vi "Begin.vi"(8 "error in":errorcluster) -> (0 "error out":errorcluster)   [LabVIEW 2015]
doc: "Called before other user functions, this VI is expected to open initial I/O refnums, load in file data, and do all program initialization. Notice that the <B>error out</B> terminal is simply used for data flow. Wiring it to other structures or subVIs ensures that this VI runs first."
uses:
  <vilib>/Rock Robotics/WPI/DriverStation/WPI_DriverStationRobotMode2.ctl
  <vilib>/Rock Robotics/WPI/Joystick/WPI_JoystickDeviceEnum.ctl
  <vilib>/Rock Robotics/SystemInterfaces/DIO/FPGA_DIOChannel.ctl
  <vilib>/Rock Robotics/WPI/Solenoid/WPI_SolenoidChannel.ctl
  Robot Global Data.vi
  <vilib>/Rock Robotics/Network Tables/NT Write String Array.vi
  <vilib>/Rock Robotics/WPI/RobotDrive/WPI_RobotDriveOpen2MotorWithCANTalonSRX.vi
  <vilib>/Rock Robotics/WPI/Utilities/WPI_GetSetVariantRefNum.vi
  <vilib>/Rock Robotics/WPI/MotorControl/WPI_MotorControlOpenCANTalonSRX.vi
  <vilib>/Rock Robotics/WPI/Solenoid/WPI_SolenoidOpenSingle.vi
  <vilib>/Rock Robotics/WPI/Solenoid/WPI_SolenoidOpenDouble.vi
  <vilib>/Rock Robotics/WPI/RobotDrive/WPI_RobotDriveOpen4MotorWithCANTalonSRX.vi
  <vilib>/Rock Robotics/WPI/Accelerometer/InternalAccelerometer/WPI_AccelerometerInternalOpen.vi
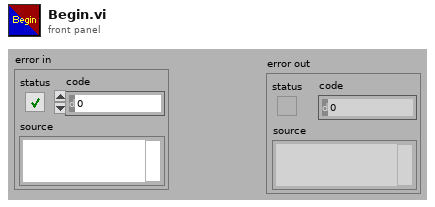
[diagram p1: front panel]
types:
  T1 = typedef "WPI_SolenoidChannel.ctl" = enum8{"Solenoid 0", "Solenoid 1", "Solenoid 2", "Solenoid 3", "Solenoid 4", "Solenoid 5", "Solenoid 6", "Solenoid 7", "Invalid"}
  T2 = typedef "FPGA_DIOChannel.ctl" = enum8{"DIO 0", "DIO 1", "DIO 2", "DIO 3", "DIO 4", "DIO 5", "DIO 6", "DIO 7", "DIO 8", "DIO 9", "DIO MXP 0", "DIO MXP 1", "DIO MXP 2", "DIO MXP 3", "DIO MXP 4", "DIO MXP 5", "DIO MXP 6", "DIO MXP 7", "DIO MXP 8", "DIO MXP 9", "DIO MXP 10", "DIO MXP 11", "DIO MXP 12", "DIO MXP 13", "DIO MXP 14", "DIO MXP 15", "Invalid"}
  T3 = typedef "WPI_JoystickDeviceEnum.ctl" = enum16{"USB 0", "USB 1", "USB 2", "USB 3", "USB 4", "USB 5"}
  T4 = typedef "WPI_DriverStationRobotMode2.ctl" = enum16{"Autonomous Disabled", "Autonomous Enabled", "Teleop Disabled", "Teleop Enabled", "Disconnected", "Finish", "Test Disabled", "Test Enabled", "Emergency Stopped"}
  T5 = typedef "WPI_AccelerometerDevRef.ctl" = cluster{"DevStatus":errorcluster, "Scaling":T6, "Analog Channels":T7, "I2C Bus":T9, "SPI Bus":T10, "Accel Range":T11, "ADXL Axes":T12, "Handle":i32, "Device Address":u8, "Accel Type":enum16{"Analog", "ADXL345 I2C", "ADXL345 SPI", "Internal", "ADXL362 SPI"}}
  T6 = typedef "WPI_AccelerometerScaling.ctl" = cluster{"Gain (VoltsPerG)":dbl, "Center Voltage":dbl}
  T7 = typedef "WPI_AccelerometerAnalogChannels.ctl" = cluster{"X-Axis":T8, "Y-Axis":T8, "Z-Axis":T8}
  T8 = typedef "FPGA_AIChannel.ctl" = enum8{"AI 0", "AI 1", "AI 2", "AI 3", "AI MXP 0", "AI MXP 1", "AI MXP 2", "AI MXP 3", "Invalid"}
  T9 = typedef "i2c_bus.ctl" = enum16{"I2C On-Board", "I2C MXP", "Invalid"}
  T10 = typedef "spi_bus.ctl" = enum16{"SPI On-Board, CS0", "SPI On-Board, CS1", "SPI On-Board, CS2", "SPI On-Board, CS3", "SPI MXP", "Invalid"}
  T11 = typedef "ADXL345 Range.ctl" = u8
  T12 = typedef "WPI_AccelerometerADXL345 Axes.ctl" = cluster{"X-Axis":bool, "Y-Axis":bool, "Z-Axis":bool}
  T13 = typedef "WPI_CompressorDevRef.ctl" = cluster{"DevStatus":errorcluster, "Pneumatics Control Module":u8}
  T14 = typedef "WPI_RobotDriveDevRef.ctl" = cluster{"DevStatus":errorcluster, "Motors[]":T15[], "Square Inputs":bool, "Max Output":dbl}
  T15 = typedef "WPI_MotorControlDeviceRef.ctl" = cluster{"DeviceStatus":errorcluster, "Type":T16, "PWM":cluster{"PWM Channel":T17, "DeadBand":T18}, "CAN":cluster{"Device Number":u8, "Control Mode":T19, "Semaphore":T20, "Max Vout":dbl, "TalonSRX Control Mode":T21}, "Invert":bool}
  T16 = typedef "WPI_MotorControlType.ctl" = enum16{"PWM", "CAN", "CANTalonSRX"}
  T17 = typedef "FPGA_DIOPWMChannel.ctl" = enum8{"PWM 0", "PWM 1", "PWM 2", "PWM 3", "PWM 4", "PWM 5", "PWM 6", "PWM 7", "PWM 8", "PWM 9", "PWM MXP 0", "PWM MXP 1", "PWM MXP 2", "PWM MXP 3", "PWM MXP 4", "PWM MXP 5", "PWM MXP 6", "PWM MXP 7", "PWM MXP 8", "PWM MXP 9", "Invalid"}
  T18 = typedef "WPI_PWMDeadband.ctl" = cluster{"Name":string, "maxPositivePwm":i32, "minPositivePwm":i32, "centerPwm":i32, "maxNegativePwm":i32, "minNegativePwm":i32, "angularRange":u16}
  T19 = typedef "WPI_CANJaguar_ControlMode.ctl" = enum8{"Percent VBus", "Current", "Speed", "Position", "Voltage"}
  T20 = typedef "Semaphore RefNum" = refnum<k1>
  T21 = typedef "WPI_CANTalonSRX_APIControlMode.ctl" = enum8{"Percent VBus", "Speed", "Position", "Slave", "Unchanged / Invalid", "Voltage Compensation", "Current", "Motion Profile"}
  T22 = typedef "WPI_JoystickDevRef.ctl" = cluster{"Device":T3}
  T23 = typedef "WPI_DigitalInputDevRef.ctl" = cluster{"DevStatus":errorcluster, "DIO Channel":T2}
  T24 = typedef "WPI_SolenoidDevRef.ctl" = cluster{"DevStatus":errorcluster, "Pneumatics Control Module":u8, "Forward Solenoid Channel":T1, "Reverse Solenoid Channel":T1}
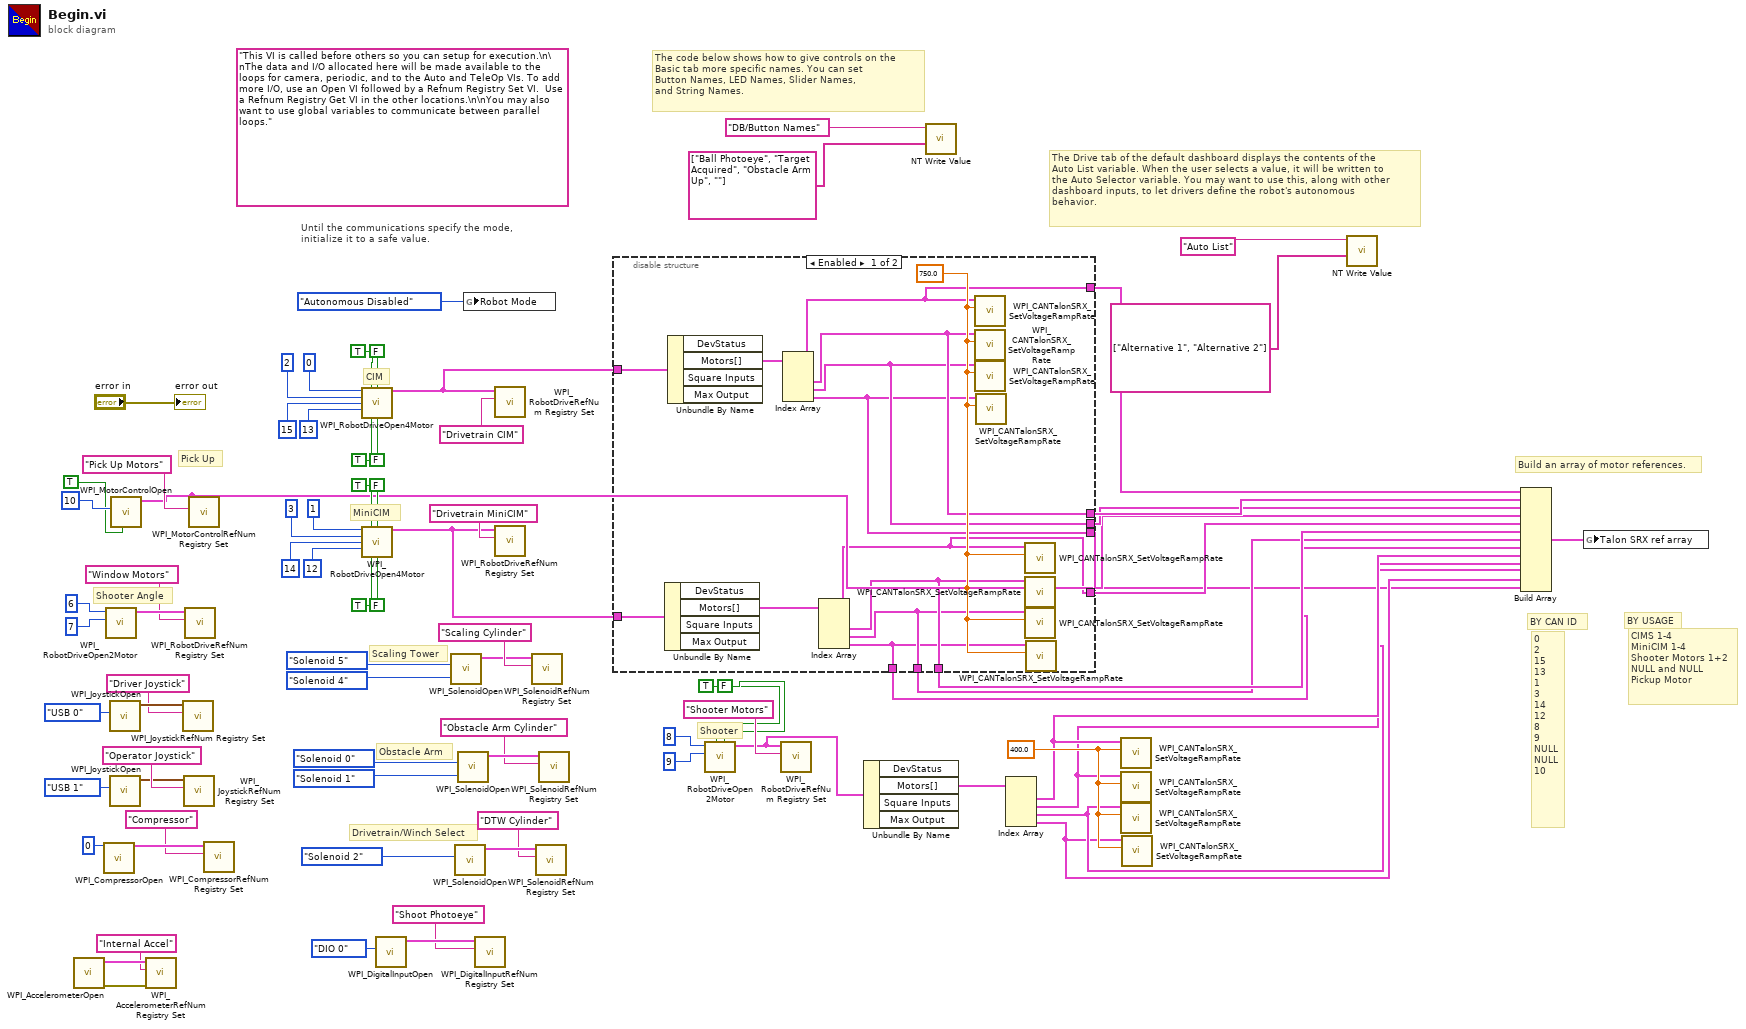
[diagram p0: block diagram]
diagram:
  w19 = 400.0
  (unwired) "This VI is called before others so you can setup for execution.\n\nThe data and I/O allocated here will be made available to the loops for camera, periodic, and to the Auto and TeleOp VIs. To add more I/O, use an Open VI followed by a Refnum Registry Set VI.  Use a Refnum Registry Get VI in the other locations.\n\nYou may also want to use global variables to communicate between parallel loops."
  # "CIMS 1-4\nMiniCIM 1-4\nShooter Motors 1+2\nNULL and NULL\nPickup Motor"
  # "BY USAGE"
  # "BY CAN ID"
  # "0\n2\n15\n13\n1\n3\n14\n12\n8\n9\nNULL\nNULL\n10"
  # "Build an array of motor references."
  # "MiniCIM"
  # "CIM"
  # "Scaling Tower"
  # "Obstacle Arm"
  # "Drivetrain/Winch Select"
  # "Shooter Angle"
  # "Pick Up"
  # "Shooter"
  # "The Drive tab of the default dashboard displays the contents of the\nAuto List variable. When the user selects a value, it will be written to\nthe Auto Selector variable. You may want to use this, along with other\ndashboard inputs, to let drivers define the robot's autonomous\nbehavior."
  # "The code below shows how to give controls on the\nBasic tab more specific names. You can set\nButton Names, LED Names, Slider Names,\nand String Names."
  # "Until the communications specify the mode,\ninitialize it to a safe value."
  n1 = call-poly <vilib>:"WPI_AccelerometerOpen.vi"() -> ("error out"=w1:errorcluster, "AccelerometerDevRef"=w3:T5)  [unwired: 10 in]
  n2 = call <vilib>:"WPI_CompressorOpen.vi"("Pneumatics Control Module (0)"=u8 0) -> ("CompressorDevRef"=w60:T13)  [unwired: 13 in, 1 out]
  n3 = call-poly <vilib>:"WPI_RobotDriveOpen2Motor.vi"("Right Motor"=u8 7, "Left Motor"=u8 6) -> ("RobotDriveDevRef"=w68:T14)  [unwired: 8 in, 1 out]
  n4 = call <vilib>:"WPI_JoystickOpen.vi"("JoystickDevice"=WPI_JoystickDeviceEnum."USB 0") -> ("JoystickDevRef"=w66:T22)  [unwired: 10 in]
  n5 = call <vilib>:"WPI_JoystickOpen.vi"("JoystickDevice"=WPI_JoystickDeviceEnum."USB 1") -> ("JoystickDevRef"=w76:T22)  [unwired: 10 in]
  n6 = call-poly <vilib>:"WPI_MotorControlOpen.vi"("Invert"=TRUE ("Left Motor Inverted"), "Device Number"=u8 10 ("Left Motor")) -> ("MotorControlDeviceRef"=w5:T15)  [unwired: 8 in, 1 out]
  n7 = call <vilib>:"WPI_AccelerometerRefNum Registry Set.vi"("error in (no error)"=w1, "refnum name"="Internal Accel", "AccelerometerDevRef"=w3) -> ()  [unwired: 7 in, 2 out]
  n8 = call <vilib>:"WPI_JoystickRefNum Registry Set.vi"("refnum name"="Driver Joystick", "JoystickDevRef"=w66) -> ()  [unwired: 8 in, 2 out]
  n9 = call <vilib>:"WPI_JoystickRefNum Registry Set.vi"("refnum name"="Operator Joystick", "JoystickDevRef"=w76) -> ()  [unwired: 8 in, 2 out]
  n10 = call <vilib>:"WPI_RobotDriveRefNum Registry Set.vi"("refnum name"="Window Motors", "RobotDriveDevRef"=w68) -> ()  [unwired: 8 in, 2 out]
  n11 = call <vilib>:"WPI_MotorControlRefNum Registry Set.vi"("refnum name"="Pick Up Motors", "MotorControlDevRef"=w5) -> ()  [unwired: 8 in, 2 out]
  n12 = call <vilib>:"WPI_CompressorRefNum Registry Set.vi"("refnum name"="Compressor", "CompressorDevRef"=w60) -> ()  [unwired: 8 in, 2 out]
  n13 = call-poly <vilib>:"WPI_RobotDriveOpen4Motor.vi"("Rear Left Motor"=u8 0, "Rear Left Motor Inverted"=TRUE, "Rear Right Motor Inverted"=FALSE, "Rear Right Motor"=u8 2, "Front Left Motor"=u8 15, "Front Right Motor"=u8 13, "Front Left Motor Inverted"=TRUE, "Front Right Motor Inverted"=FALSE) -> ("RobotDriveDevRef"=w23:T14)  [unwired: 6 in, 1 out]
  n14 = call-poly <vilib>:"WPI_RobotDriveOpen4Motor.vi"("Rear Left Motor"=u8 1, "Rear Left Motor Inverted"=TRUE, "Rear Right Motor Inverted"=FALSE, "Rear Right Motor"=u8 3, "Front Left Motor"=u8 14, "Front Right Motor"=u8 12, "Front Left Motor Inverted"=TRUE, "Front Right Motor Inverted"=FALSE) -> ("RobotDriveDevRef"=w22:T14)  [unwired: 6 in, 1 out]
  n15 = call <vilib>:"WPI_DigitalInputOpen.vi"("DIO Channel"=FPGA_DIOChannel."DIO 0") -> ("DigitalInputDevRef"=w62:T23)  [unwired: 9 in, 1 out]
  n16 = call-poly <vilib>:"WPI_SolenoidOpen.vi"("Reverse Solenoid Channel"=WPI_SolenoidChannel."Solenoid 5", "Forward Solenoid Channel"=WPI_SolenoidChannel."Solenoid 4") -> ("SolenoidDevRef"=w44:T24)  [unwired: 8 in, 1 out]
  n17 = call-poly <vilib>:"WPI_SolenoidOpen.vi"("Solenoid Channel"=WPI_SolenoidChannel."Solenoid 2" ("Forward Solenoid Channel")) -> ("SolenoidDevRef"=w54:T24)  [unwired: 9 in, 1 out]
  n18 = call-poly <vilib>:"WPI_SolenoidOpen.vi"("Reverse Solenoid Channel"=WPI_SolenoidChannel."Solenoid 0", "Forward Solenoid Channel"=WPI_SolenoidChannel."Solenoid 1") -> ("SolenoidDevRef"=w49:T24)  [unwired: 8 in, 1 out]
  n19 = global write "Robot Global Data.vi" "Robot Mode"(WPI_DriverStationRobotMode2."Autonomous Disabled" ("Robot Mode")) -> ()
  n20 = call <vilib>:"WPI_DigitalInputRefNum Registry Set.vi"("refnum name"="Shoot Photoeye", "DigitalInputDevRef"=w62) -> ()  [unwired: 8 in, 2 out]
  n21 = call <vilib>:"WPI_RobotDriveRefNum Registry Set.vi"("refnum name"="Drivetrain CIM", "RobotDriveDevRef"=w23) -> ()  [unwired: 8 in, 2 out]
  n22 = call <vilib>:"WPI_RobotDriveRefNum Registry Set.vi"("refnum name"="Drivetrain MiniCIM", "RobotDriveDevRef"=w22) -> ()  [unwired: 8 in, 2 out]
  n23 = call <vilib>:"WPI_SolenoidRefNum Registry Set.vi"("refnum name"="Scaling Cylinder", "SolenoidDevRef"=w44) -> ()  [unwired: 8 in, 2 out]
  n24 = call <vilib>:"WPI_SolenoidRefNum Registry Set.vi"("refnum name"="DTW Cylinder", "SolenoidDevRef"=w54) -> ()  [unwired: 8 in, 2 out]
  n25 = call <vilib>:"WPI_SolenoidRefNum Registry Set.vi"("refnum name"="Obstacle Arm Cylinder", "SolenoidDevRef"=w49) -> ()  [unwired: 8 in, 2 out]
  n26 = disable-structure shown="Enabled" {
    disable-tunnel: w23 -> [w94 _]
    disable-tunnel: w22 -> [w91 _]
    disable-tunnel: [w89 _] -> w17
    disable-tunnel: [w88 _] -> w16
    disable-tunnel: [w87 _] -> w15
    disable-tunnel: [w86 _] -> w14
    disable-tunnel: [w85 _] -> w13
    disable-tunnel: [w84 _] -> w12
    disable-tunnel: [w83 _] -> w11
    disable-tunnel: [w82 _] -> w10
    frame Enabled {
      w90 = 750.0
      n27 = Unbundle By Name(w91) -> ("Motors[]"=w92:T15[])  [unwired: 3 out]
      n28 = Unbundle By Name(w94) -> ("Motors[]"=w93:T15[])  [unwired: 3 out]
      n29 = Index Array(array=w93) -> (element #1=w89:T15, element #2=w88:T15, element #3=w87:T15, element #4=w86:T15)  [unwired: 4 in]
      n30 = Index Array(array=w92) -> (element #1=w85:T15, element #2=w84:T15, element #3=w83:T15, element #4=w82:T15)  [unwired: 4 in]
      n31 = call <vilib>:"WPI_CANTalonSRX_SetVoltageRampRate.vi"("Throttle Ramp Rate (percent/s)"=w90, "CAN Talon SRX Ref"=w89) -> ()  [unwired: 8 in, 2 out]
      n32 = call <vilib>:"WPI_CANTalonSRX_SetVoltageRampRate.vi"("Throttle Ramp Rate (percent/s)"=w90, "CAN Talon SRX Ref"=w88) -> ()  [unwired: 8 in, 2 out]
      n33 = call <vilib>:"WPI_CANTalonSRX_SetVoltageRampRate.vi"("Throttle Ramp Rate (percent/s)"=w90, "CAN Talon SRX Ref"=w87) -> ()  [unwired: 8 in, 2 out]
      n34 = call <vilib>:"WPI_CANTalonSRX_SetVoltageRampRate.vi"("Throttle Ramp Rate (percent/s)"=w90, "CAN Talon SRX Ref"=w86) -> ()  [unwired: 8 in, 2 out]
      n35 = call <vilib>:"WPI_CANTalonSRX_SetVoltageRampRate.vi"("Throttle Ramp Rate (percent/s)"=w90, "CAN Talon SRX Ref"=w85) -> ()  [unwired: 8 in, 2 out]
      n36 = call <vilib>:"WPI_CANTalonSRX_SetVoltageRampRate.vi"("Throttle Ramp Rate (percent/s)"=w90, "CAN Talon SRX Ref"=w84) -> ()  [unwired: 8 in, 2 out]
      n37 = call <vilib>:"WPI_CANTalonSRX_SetVoltageRampRate.vi"("Throttle Ramp Rate (percent/s)"=w90, "CAN Talon SRX Ref"=w83) -> ()  [unwired: 8 in, 2 out]
      n38 = call <vilib>:"WPI_CANTalonSRX_SetVoltageRampRate.vi"("Throttle Ramp Rate (percent/s)"=w90, "CAN Talon SRX Ref"=w82) -> ()  [unwired: 8 in, 2 out]
    }
    frame Disabled {
    }
  }
  n39 = call-poly <vilib>:"WPI_RobotDriveOpen2Motor.vi"("Right Motor Inverted"=FALSE, "Left Motor Inverted"=TRUE, "Right Motor"=u8 9, "Left Motor"=u8 8) -> ("RobotDriveDevRef"=w21:T14)  [unwired: 6 in, 1 out]
  n40 = call <vilib>:"WPI_RobotDriveRefNum Registry Set.vi"("refnum name"="Shooter Motors", "RobotDriveDevRef"=w21) -> ()  [unwired: 8 in, 2 out]
  n41 = Unbundle By Name(w21) -> ("Motors[]"=w20:T15[])  [unwired: 3 out]
  n42 = call-poly <vilib>:"NT Write Value.vi"("String Array"=string[] ["Ball Photoeye", "Target Acquired", "Obstacle Arm Up", ""], "Name"="DB/Button Names") -> ()  [unwired: 9 in, 1 out]
  n43 = Index Array(array=w20) -> (element #1=w9:T15, element #2=w8:T15, element #3=w7:T15, element #4=w6:T15)  [unwired: 4 in]
  n44 = call <vilib>:"WPI_CANTalonSRX_SetVoltageRampRate.vi"("Throttle Ramp Rate (percent/s)"=w19, "CAN Talon SRX Ref"=w9) -> ()  [unwired: 8 in, 2 out]
  n45 = call <vilib>:"WPI_CANTalonSRX_SetVoltageRampRate.vi"("Throttle Ramp Rate (percent/s)"=w19, "CAN Talon SRX Ref"=w8) -> ()  [unwired: 8 in, 2 out]
  n46 = call <vilib>:"WPI_CANTalonSRX_SetVoltageRampRate.vi"("Throttle Ramp Rate (percent/s)"=w19, "CAN Talon SRX Ref"=w7) -> ()  [unwired: 8 in, 2 out]
  n47 = call <vilib>:"WPI_CANTalonSRX_SetVoltageRampRate.vi"("Throttle Ramp Rate (percent/s)"=w19, "CAN Talon SRX Ref"=w6) -> ()  [unwired: 8 in, 2 out]
  n48 = call-poly <vilib>:"NT Write Value.vi"("String Array"=string[] ["Alternative 1", "Alternative 2"], "Name"="Auto List") -> ()  [unwired: 9 in, 1 out]
  n49 = Build Array(w17, w16, w15, w14, w13, w12, w11, w10, w9, w8, w7, w6, w5) -> (w4:T15[])
  n50 = global write "Robot Global Data.vi" "Talon SRX ref array"(w4) -> ()
  "error out" <- "error in"
